vi "ProgramInitialStep.vi"(8 "error in (no error)":errorcluster, 11 "RealWorkActor in":refnum<class "RealWorkActor.lvclass">) -> (0 "error out":errorcluster, 3 "RealWorkActor out":refnum<class "RealWorkActor.lvclass">)   [LabVIEW 2014, in "RealWorkActor.lvclass"]
uses:
  RealWorkActor.lvclass
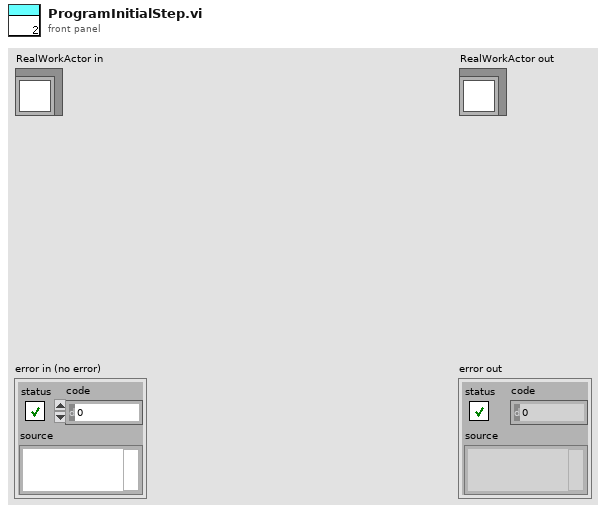
[diagram p1: front panel]
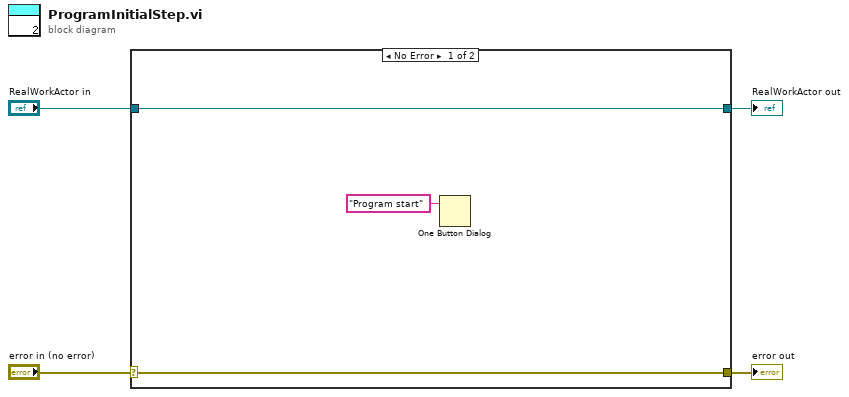
[diagram p0: block diagram]
diagram:
  n1 = case shown="No Error" "error in (no error)" {
    selector: "error in (no error)" -> [w7 w9]
    tunnel: [w7 w9] -> w3
    tunnel: [w6 w8] -> w1
    tunnel: "RealWorkActor in" -> [w6 w8]
    frame No Error {
      n2 = One Button Dialog(message="Program start") -> ()  [unwired: 1 in, 1 out]
    }
    frame Error {
    }
  }
  "error out" <- w3
  "RealWorkActor out" <- w1
